vi "Load Image From Memory.vi"(8 "error in (no error)":errorcluster, 11 "Encoded Image":u8[](array[numeric])) -> (0 "error out":errorcluster, 2 "Image":T1)   [LabVIEW 2020, in "G-Image.lvlib"]
doc: "Decodes the byte array to a LabVIEW picture."
uses:
  G-Image.lvlib
  <vilib>/picture/picture.llb/imagedata.ctl
  Private/RGBA To ARGB.vi
  <vilib>/Utility/error.llb/Error Cluster From Error Code.vi
  <vilib>/picture/picture.llb/Create Mask By Alpha.vi
  lib/g_image_32.dll
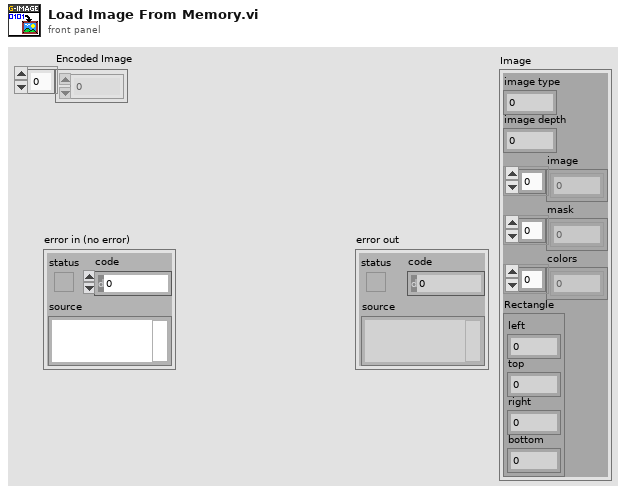
[diagram p1: front panel]
types:
  T1 = typedef "imagedata.ctl" = cluster{"image type":i32, "image depth":i32, "image":u8[], "mask":u8[], "colors":u32[], "Rectangle":cluster{"left":i16, "top":i16, "right":i16, "bottom":i16}}
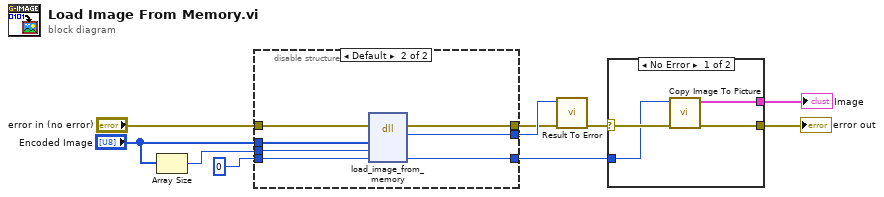
[diagram p0: block diagram]
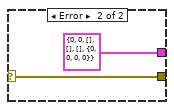
[diagram p2: hidden frame]
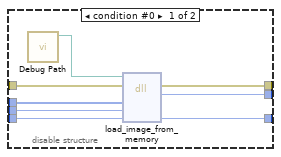
[diagram p3: hidden frame]
diagram:
  n1 = Array Size(array="Encoded Image") -> (size(s)=w1:i32)
  n2 = disable-structure shown="Default" {
    disable-tunnel: [w17 w25] -> w7
    disable-tunnel: "error in (no error)" -> [w16 w24]
    disable-tunnel: "Encoded Image" -> [w15 w23]
    disable-tunnel: [w14 w22] -> w8
    disable-tunnel: [w13 w20] -> w4
    disable-tunnel: i64 0 ("count") -> [w12 w21]
    disable-tunnel: w1 -> [w11 w19]
    frame condition #0 {
      n3 = call "Debug Path.vi"() -> ("Debug Path"=w18:path)  [unwired: 11 in]
      n4 = dll-call lib="?" fn="load_image_from_memory"(path in=w18, error in=w16, "encoded_image"=w15, "encoded_image_size"=w11, "image_out"=w12) -> (error out=w17:errorcluster, "result"=w14:i32, "image_out"=w13:i64)  [unwired: 3 in, 1 out]
    }
    frame condition #1 (active) {
      n5 = dll-call lib="C:/github/dataflowg/g-image/src/LabVIEW/G-Image/lib/g_image_*.*" fn="load_image_from_memory"(error in=w24, "encoded_image"=w23, "encoded_image_count"=w19, "image_out"=w21) -> (error out=w25:errorcluster, "result"=w22:i32, "image_out"=w20:i64)  [unwired: 4 in, 1 out]
    }
  }
  n6 = call "Result To Error.vi"("error in (no error)"=w7, "Result Code"=w8) -> ("error out"=w6:errorcluster)  [unwired: 9 in]
  n7 = case shown="No Error" w6 {
    selector: w6 -> [w29 w31]
    tunnel: [w27 w31] -> w10
    tunnel: w4 -> [w28 _]
    tunnel: [w26 T1 {"image type"=0, "image depth"=0, "image"=[], "mask"=[], "colors"=[], "Rectangle"={"left"=0, "top"=0, "right"=0, "bottom"=0}} ("Image")] -> w3
    frame No Error {
      n8 = call "Copy Image To Picture.vi"("error in (no error)"=w29, "image_ptr"=w28) -> ("error out"=w27:errorcluster, "Image"=w26:T1)  [unwired: 8 in]
    }
    frame Error {
    }
  }
  "error out" <- w10
  "Image" <- w3
